vi "ReadIVIsampleDMM.vi"(0 "instrument handle":refnum<k15>, 1 "error in (no error)":errorcluster) -> (2 "instrument handle out":refnum<k15>, 3 "Waveform Chart":dbl(graph), 4 "Array":dbl[](array[numeric]) format="%.2f", 5 "error out":errorcluster)   [LabVIEW 2012]
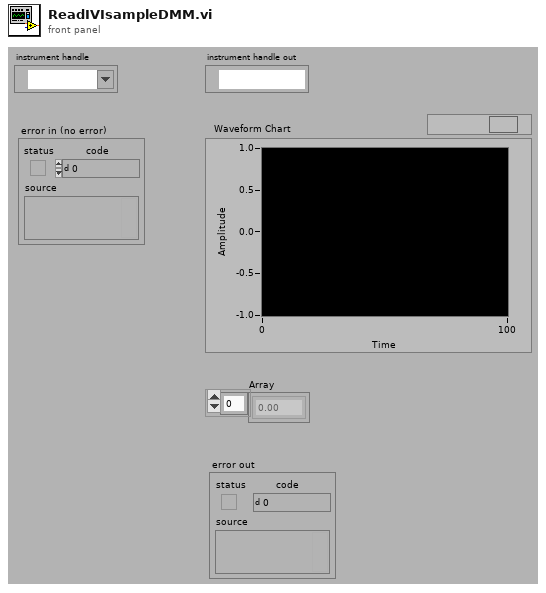
[diagram p1: front panel]
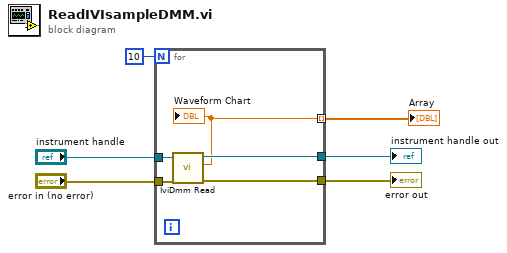
[diagram p0: block diagram]
diagram:
  n1 = for {
    N: 10 -> [_]
    tunnel: "instrument handle" -> [w11]
    tunnel: "error in (no error)" -> [w10]
    tunnel: [w9] -> w3
    tunnel: [w8] -> w4
    tunnel: [w7] -> w6 mode=indexing
    n2 = call <vilib>:"IviDmm Read.vi"("error in (no error)"=w10, "instrument handle"=w11) -> ("error out"=w8:errorcluster, "reading"=w7:dbl, "instrument handle out"=w9:refnum<k15>)  [unwired: 1 in, 6 out]
    "Waveform Chart" <- w7
  }
  "Array" <- w6
  "error out" <- w4
  "instrument handle out" <- w3
